vi "MAIN - TLB` Springboard Tool.vi"() -> ()   [LabVIEW 2015, in "TLB` Springboard.lvlib"]
doc: "TLB Prime - Application Template 1.3.0.24\nNorm Kirchner, NI Systems Engineering - NI\nCopyright (c) 2014, NI"
uses:
  TLB` Springboard.lvlib
  Components/State Declaration.ctl
  Components/System Triggers.ctl
  <vilib>/Utility/error.llb/DialogTypeEnum.ctl
  <vilib>/NI/AMC/Read Termination Message.vi
  <vilib>/NI/AMC/Create Single Message.vi
  <vilib>/NI/AMC/Update Message Routing Info.vi
  <vilib>/NI/AMC/Create Multiple Messages.vi
  Components/TypeDef - SHIFTER - TLB` Springboard.ctl
  <vilib>/NI/AMC/Globals.vi
  <vilib>/NI/AMC/Send Message.vi
  Components/Dependencies.llb/TLB`_Dependencies.lvlib
  <vilib>/NI/AMC/AMC.lvlib
panel:
  in  "Tab Control":T1(tab)
  out "Application:All Libraries in Application Instance":string[](array[string])
  out "Owned Items[]":refnum<vi>[](array[refnum])
  out "Array 1":string[](array[string])
  out "Array 2":string[](array[string])
  out "size(s) 1":i32
  out "size(s) 2":i32
  out "size(s) 4":i32
  out "Array 3":string[](array[string])
  out "Array 4":string[](array[string])
  out "Array 6":string[](array[string])
  out "Array 5":string[](array[string])
  out "size(s) 6":i32
  in  "Library Path":path=path "C:/Repositories/TLB-Prime/Source/TLB' Template 2/TLB` Template/TLB` Template.lvlib"
  in  "Add to Project":u16(ring) items=["< Create In New Project... >"]
  in  "Cancel":bool
  in  "Build":bool
  in  "New TLB Name":string="TEST"
  in  "Destination Folder":path=path "C:/Repositories/TLB-Prime/Stage"
  out "error out":errorcluster
  # "TLB` Springboard"
  # "Description"
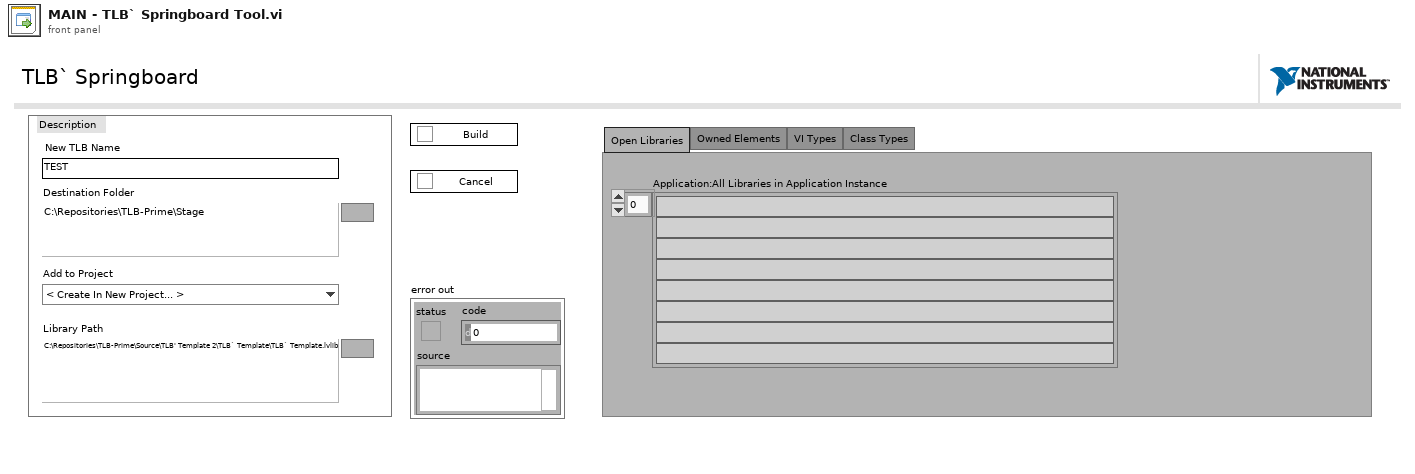
[diagram p1: front panel]
types:
  T1 = enum32{"Open Libraries", "Owned Elements", "VI Types", "Class Types"}
  T2 = typedef "TLB` Springboard.lvlib/System Triggers.ctl" = enum16{"<None>", "Create New", "Cache User Parameters", "Close Application"}
  T3 = typedef "TLB` Springboard.lvlib/State Declaration.ctl" = enum16{"<Startup>", "Idle", "Creating", "<Shutdown>"}
  T4 = enum16{"Clear SR", "Set Display", "Set Shifter", "Initialize Events", "Init Q"}
  T5 = typedef "TLB` Springboard.lvlib/TypeDef - SHIFTER - TLB` Springboard.ctl" = cluster{"State":T3, "User Data":cluster{"New TLB Name":string, "Destination Folder":path, "Project Selection":u16, "Library Path":path}, "Display Data":cluster{"Active Item Tag":string}, "User Parameter Controls":refnum<vi>[], "Framework Data":cluster{"Exit Event":T6, "Terminate Error":errorcluster}, "Private Data":cluster{"Projects In Memory":refnum<vi>[], "Build Complete":bool, "My Computer Ref":refnum<vi>, "Application Ref":refnum<vi>, "Library Ref":refnum<vi>, "Owned Items[]":refnum<vi>[]}}
  T6 = typedef "TLB` Springboard.lvlib/TLB`_Dependencies.lvlib/Exit Event Ref.ctl" = refnum<user-event>
  T7 = typedef "AMC.lvlib/Message Queue.ctl" = refnum<queue>
  T8 = typedef "DialogTypeEnum.ctl" = enum16{"no dialog", "OK message", "continue or stop message", "auto error handling dialog", "OK message + warnings", "continue/stop + warnings"}
  T9 = enum8{"Enabled", "Disabled", "Disabled and Grayed Out"}
  T10 = enum32{"Invalid", "Standard", "Closed", "Hidden", "Minimized", "Maximized"}
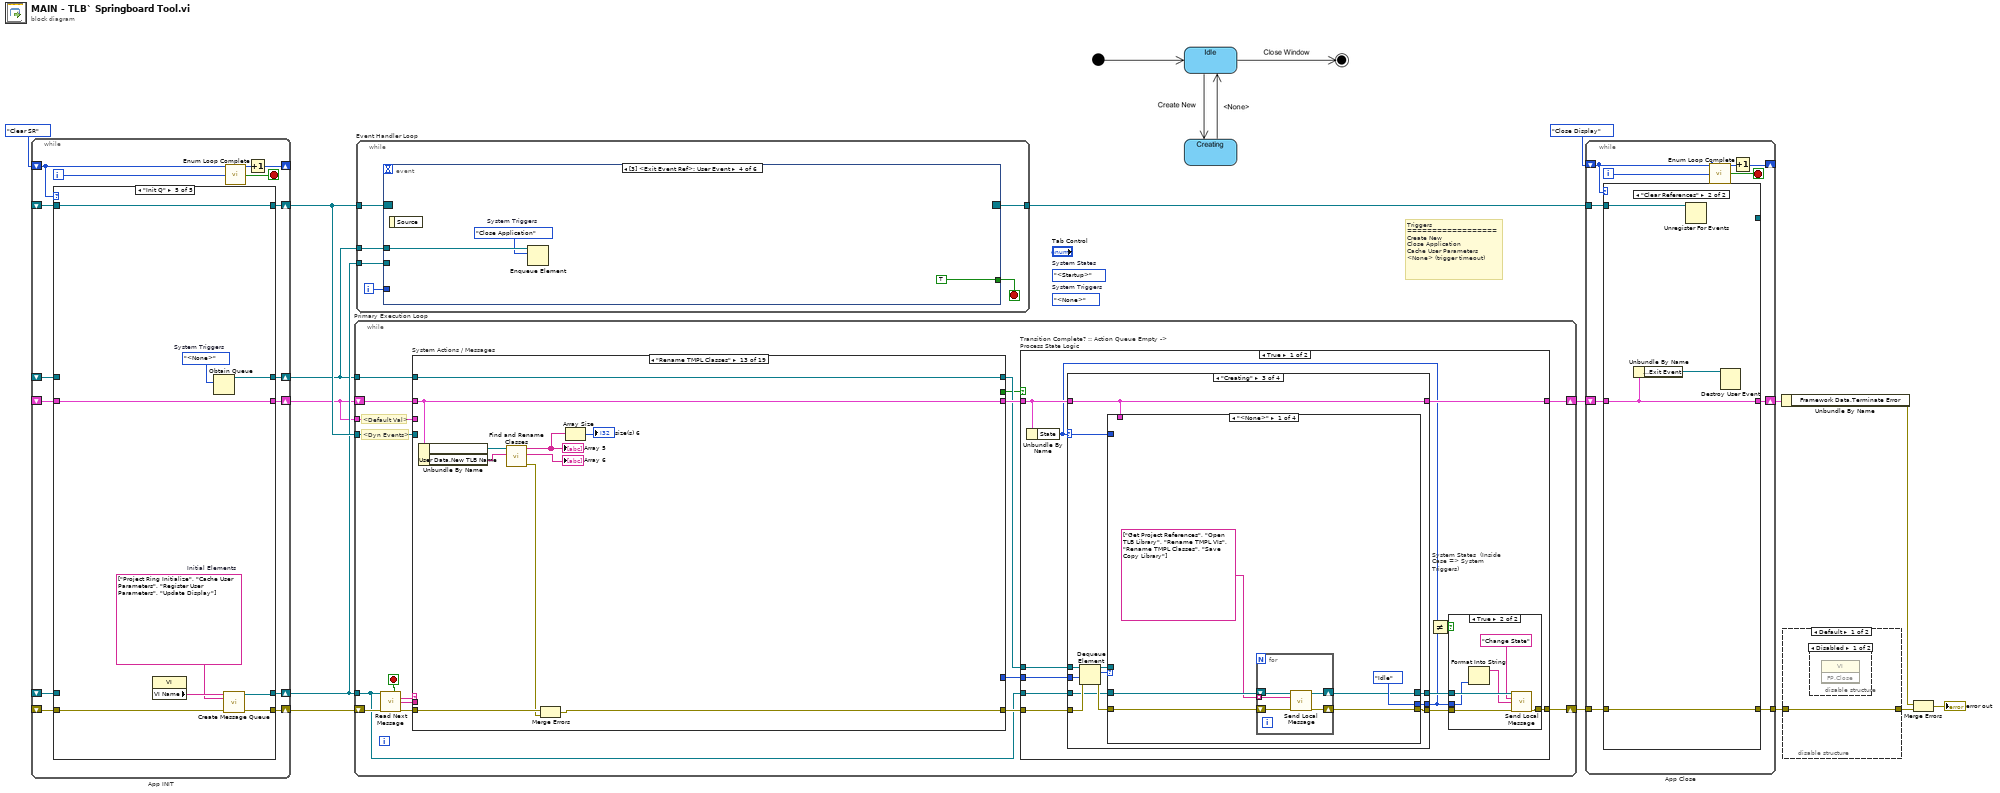
[diagram p0: block diagram]
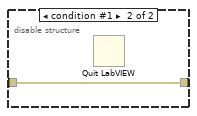
[diagram p3: hidden frame]
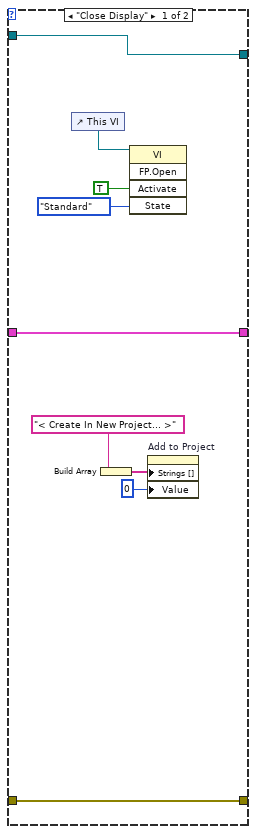
[diagram p4: hidden frame]
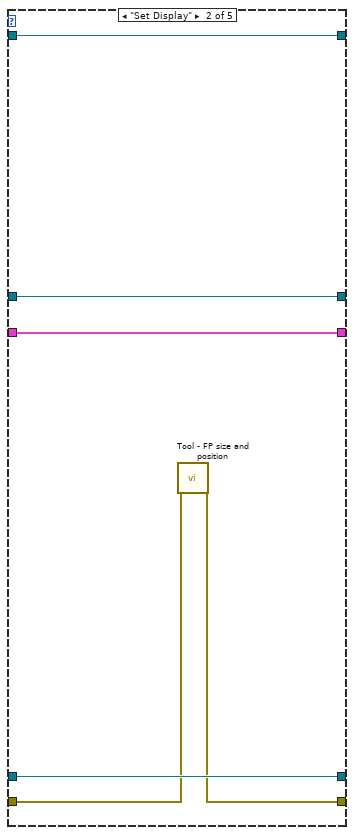
[diagram p6: hidden frame]
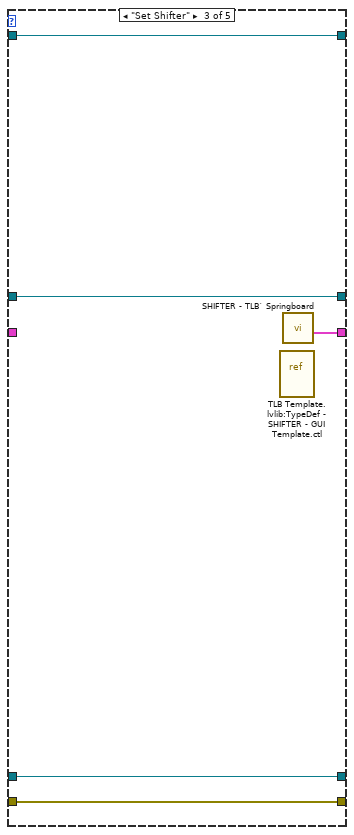
[diagram p7: hidden frame]
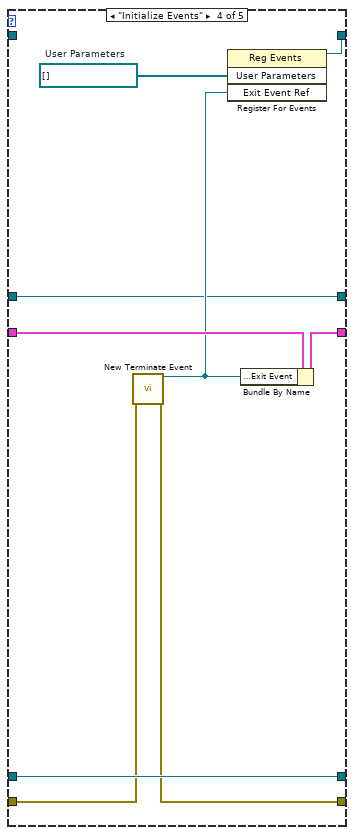
[diagram p8: hidden frame]
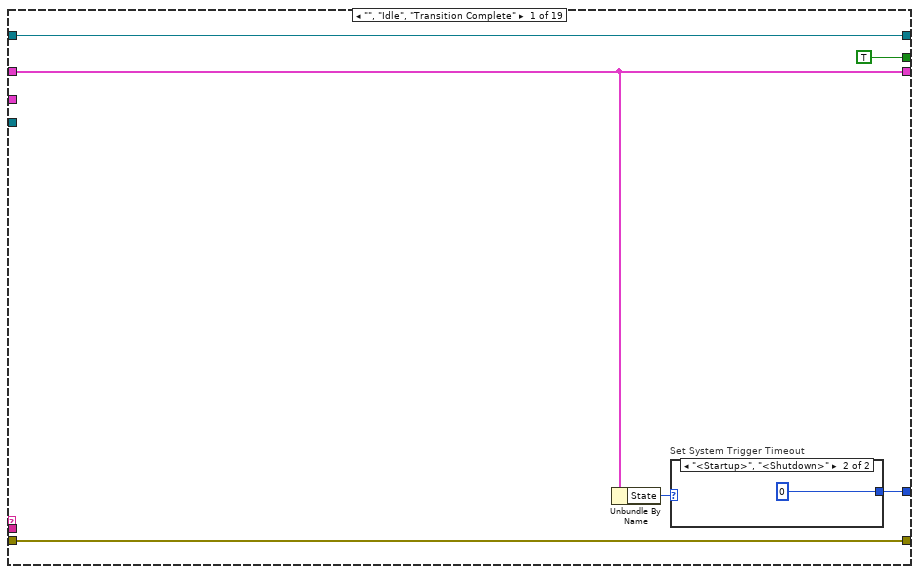
[diagram p9: hidden frame]
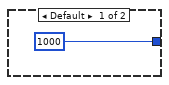
[diagram p10: hidden frame]
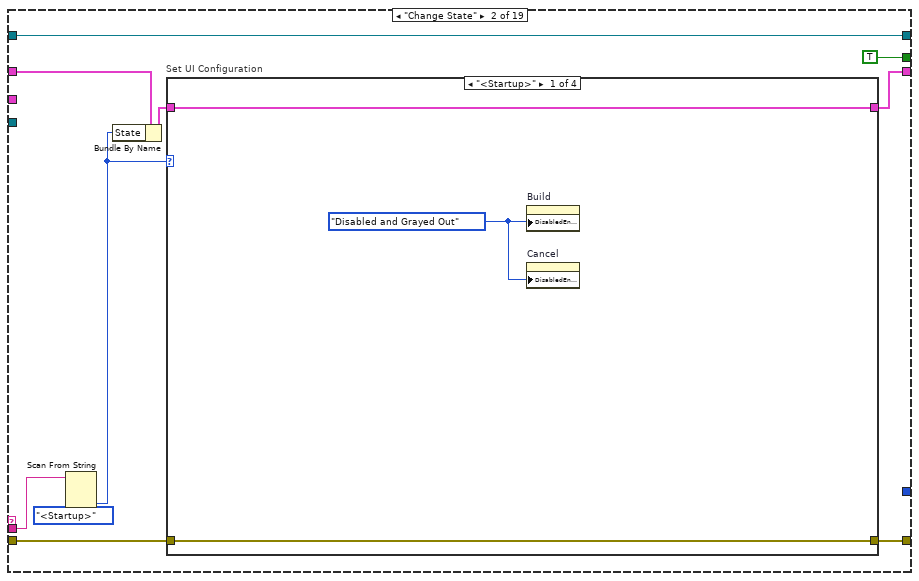
[diagram p11: hidden frame]
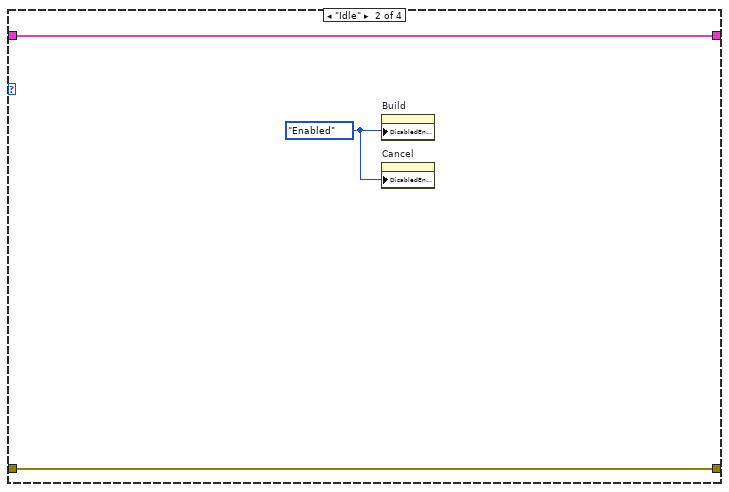
[diagram p12: hidden frame]
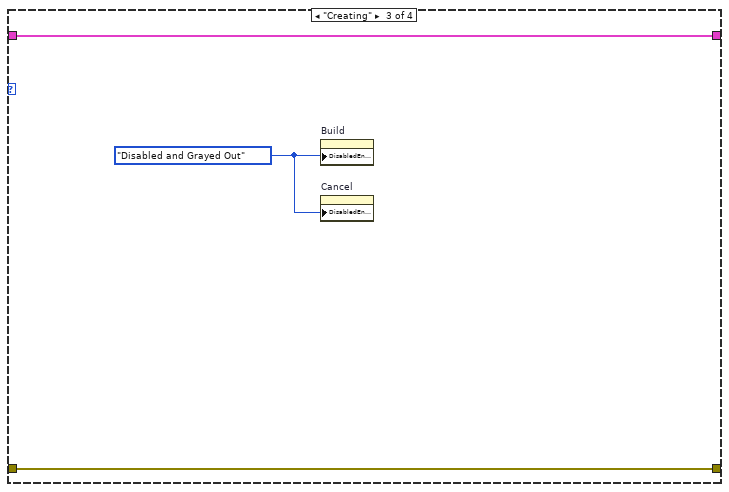
[diagram p13: hidden frame]
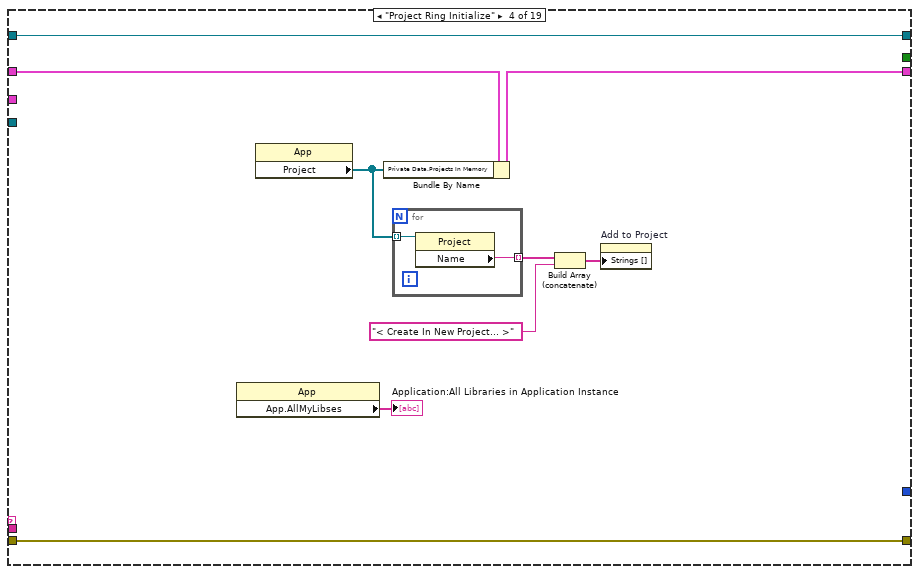
[diagram p16: hidden frame]
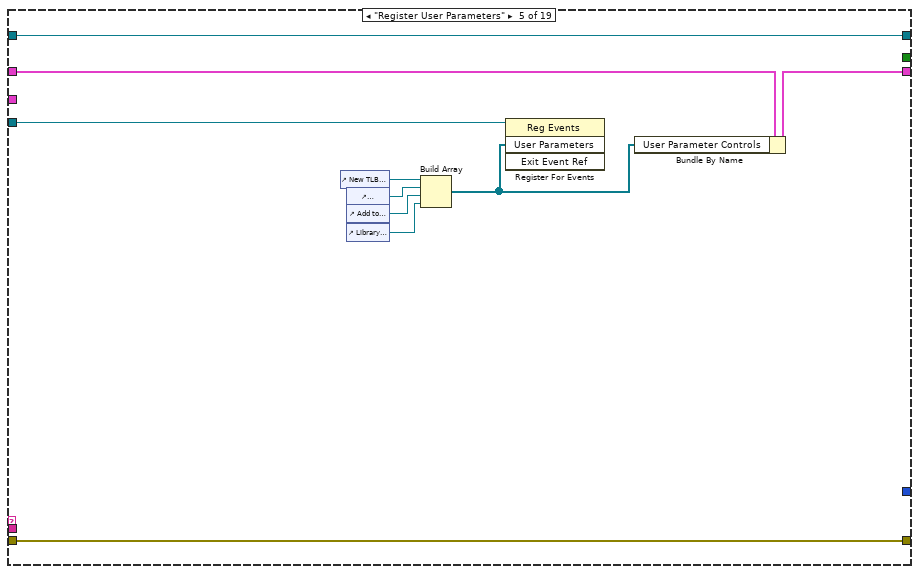
[diagram p17: hidden frame]
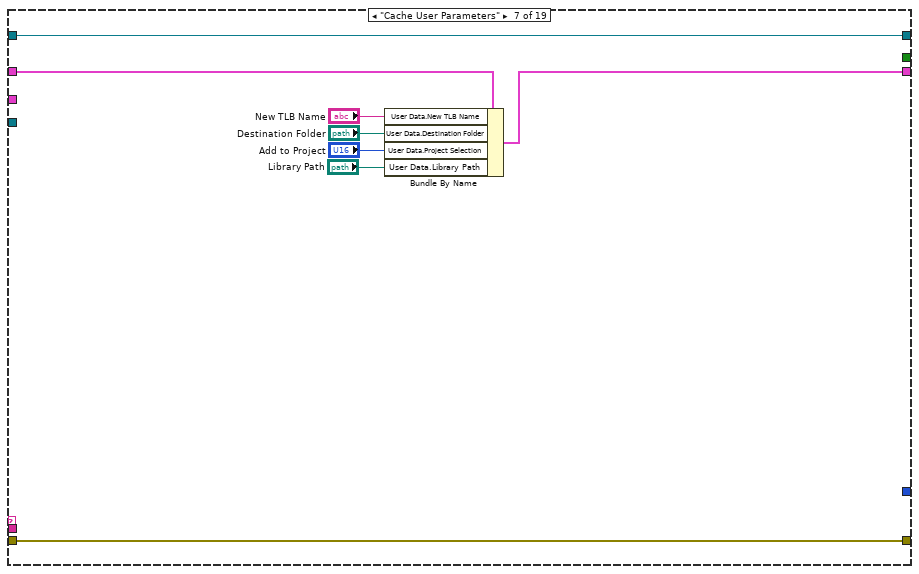
[diagram p19: hidden frame]
diagram:
  (unwired) System_Triggers."<None>"  # System Triggers
  (unwired) State_Declaration."<Startup>"  # System States
  # "Triggers\n==================\nCreate New\nClose Application\nCache User Parameters\n<None> (trigger timeout)"
  n1 = while "App INIT" {
    shift-right: [w23] -> _
    shift-left: T4."Clear SR" -> [w18]
    shift-right: [w29] -> w9
    shift-left: _ -> [w22]
    shift-right: [w26] -> w8
    shift-left: _ -> [w21]
    shift-right: [w28] -> w11
    shift-left: _ -> [w20]
    shift-right: [w27] -> w1
    shift-left: _ -> [w19]
    shift-right: [w17] -> w2
    shift-left: _ -> [w16]
    i -> [w24]
    stop <- w25 stop-if-true
    n2 = case shown="\"Init Q\"" w18 {
      tunnel: [_ w33 w40 w49 w55] -> w29
      tunnel: [_ w31 w39 w42 w53] -> w26
      tunnel: [_ w35 w36 w46 w57] -> w27
      tunnel: [_ w34 w38 w45 w58] -> w28
      tunnel: w22 -> [_ w33 w40 w49 _]
      tunnel: w21 -> [_ w32 w39 w43 w54]
      tunnel: w20 -> [_ w34 w38 _ w58]
      tunnel: w19 -> [_ w35 _ w47 w57]
      tunnel: [_ w30 w37 w41 w51] -> w17
      tunnel: w16 -> [_ w30 w37 w41 _]
      frame "Clear SR" {
      }
      frame "Set Display" {
        n3 = call "Tool - FP size and position.vi"("error in (no error)"=w32) -> ("error out"=w31:errorcluster)  [unwired: 7 in, 11 out]
      }
      frame "Set Shifter" {
        n4 = vi-ref "TLB Template.lvlib:TypeDef - SHIFTER - GUI Template.ctl"() -> ()  [unwired: 1 out]
        n5 = call "SHIFTER - TLB` Springboard.vi"() -> ("SHIFTER DATA"=w36:T5)  [unwired: 15 in]
      }
      frame "Initialize Events" {
        w48 = refnum<vi>[] []  # User Parameters
        n6 = call "New Terminate Event.vi"("error in (no error)"=w43) -> ("Exit Event Ref"=w44:T6, "error out"=w42:errorcluster)  [unwired: 13 in]
        n7 = register-events(w48, w44) -> (reference out=w45:refnum<event-registration>)  [unwired: 2 in, 1 out]
        n8 = Bundle By Name(cluster=w47, "Framework Data.Exit Event"=w44) -> (w46:T5)
      }
      frame "Init Q" {
        w50 = System_Triggers."<None>"  # System Triggers
        w52 = string[] ["Project Ring Initialize", "Cache User Parameters", "Register User Parameters", "Update Display"]  # Initial Elements
        n9 = property class="VI"() -> ("VI Name"=w56:string)  [unwired: 2 in, 2 out]
        n10 = Obtain Queue(element data type=w50) -> (queue out=w51:refnum<queue>)  [unwired: 4 in, 2 out]
        n11 = call <vilib>:"Create Message Queue.vi"("message queue name"=w56, "initial message names"=w52, "error in"=w54) -> ("message queue out"=w55:T7, "error out"=w53:errorcluster)  [unwired: 11 in]
      }
    }
    n12 = call "Enum Loop Complete.vi"("Current State Enum"=w18, "Itteration"=w24) -> ("Loop Complete?"=w25:bool)  [unwired: 13 out]
    n13 = Increment(x=w18) -> (x+1=w23:T4)
  }
  n14 = while "Primary Execution Loop" {
    shift-right: [w65] -> w15
    shift-left: w8 -> [w72]
    shift-right: [w68] -> w14
    shift-left: w1 -> [w75]
    tunnel: w1 -> [w74]
    tunnel: w9 -> [w63]
    tunnel: w11 -> [w73]
    tunnel: w2 -> [w64]
    stop <- w70 stop-if-true
    # "<Dyn Events>"
    # "<Default Val>"
    n15 = call <vilib>:"Read Next Message.vi"("message queue in"=w63, "error in"=w72) -> ("exit process?"=w70:bool, "message name"=w69:string, "message value"=w60:string, "error out"=w71:errorcluster)  [unwired: 6 in, 4 out]
    n16 = case "System Actions / Messages" shown="\"Rename TMPL Classes\"" w69 {
      selector: w69 -> [_ _ _ _ _ _ _ _ _ _ _ _ _ _ _ _ _ _ w282]
      tunnel: [w81 w88 w107 w114 w128 w131 w137 w142 w145 w157 w177 w184 w195 w220 w245 w250 w272 w276 w286] -> w66
      tunnel: w71 -> [w81 w87 w107 w114 w128 w131 w137 w142 w145 w157 w178 w192 w202 w224 w245 w251 w272 w275 w287]
      tunnel: w75 -> [w76 w84 w106 w116 w127 w130 w139 w141 w144 w150 w176 w187 w198 w219 w244 w248 w271 w279 w288]
      tunnel: w74 -> [_ _ _ _ _ _ _ _ _ _ _ _ _ _ _ _ _ _ _]
      tunnel: [w76 w86 w106 w111 w126 w130 w138 w141 w144 w148 w172 w187 w198 w218 w244 w249 w271 w279 w288] -> w67
      tunnel: [w77 _ _ _ _ _ _ _ _ _ _ _ _ _ _ _ _ _ _] -> w59
      tunnel: w73 -> [_ _ _ _ w125 _ _ _ _ _ _ _ _ _ _ _ _ _ _]
      tunnel: [w79 w92 w105 w115 w124 w129 w136 w140 w143 w156 w179 w191 w201 w225 w243 w246 w270 w273 w280] -> w62
      tunnel: w64 -> [w79 w92 w105 w115 w124 w129 w136 w140 w143 w156 w179 w191 w201 w225 w243 w246 w270 w273 w280]
      tunnel: [TRUE TRUE _ _ _ _ _ _ _ _ _ _ _ _ _ _ _ _ _] -> w61
      tunnel: w60 -> [_ w91 _ _ _ _ _ _ _ _ _ _ _ _ _ _ _ _ _]
      frame "", "Idle", "Transition Complete" {
        n17 = Unbundle By Name(w76) -> ("State"=w78:T3)
        n18 = case "Set System Trigger Timeout" shown="\"<Startup>\", \"<Shutdown>\"" w78 {
          tunnel: [1000 0] -> w77
          frame Default {
          }
          frame "<Startup>", "<Shutdown>" {
          }
        }
      }
      frame "Change State" {
        n19 = Scan From String(input string=w91, default 1=State_Declaration."<Startup>" ("State")) -> (output 1=w89:T3)  [unwired: 3 in, 3 out]
        n20 = Bundle By Name(cluster=w84, "State"=w89) -> (w85:T5)
        n21 = case "Set UI Configuration" shown="\"<Startup>\"" w89 {
          tunnel: [w95 w99 w102 w104] -> w88
          tunnel: w87 -> [w95 w99 w102 w104]
          tunnel: [w96 w98 w101 w103] -> w86
          tunnel: w85 -> [w96 w98 w101 w103]
          frame "<Startup>" {
            w94 = T9."Disabled and Grayed Out" ("Disabled")
            n22 = property on="Build" class="Bool"("DisabledEnum"=w94) -> ()  [unwired: 2 in, 2 out]
            n23 = property on="Cancel" class="Bool"("DisabledEnum"=w94) -> ()  [unwired: 2 in, 2 out]
          }
          frame "Idle" {
            w97 = T9."Enabled" ("Disabled")
            n24 = property on="Build" class="Bool"("DisabledEnum"=w97) -> ()  [unwired: 2 in, 2 out]
            n25 = property on="Cancel" class="Bool"("DisabledEnum"=w97) -> ()  [unwired: 2 in, 2 out]
          }
          frame "Creating" {
            w100 = T9."Disabled and Grayed Out" ("Disabled")
            n26 = property on="Build" class="Bool"("DisabledEnum"=w100) -> ()  [unwired: 2 in, 2 out]
            n27 = property on="Cancel" class="Bool"("DisabledEnum"=w100) -> ()  [unwired: 2 in, 2 out]
          }
          frame "<Shutdown>" {
          }
        }
      }
      frame "/***********Initialize***********/" {
      }
      frame "Project Ring Initialize" {
        n28 = property class="App"() -> ("App.AllMyLibses"=→"Application:All Libraries in Application Instance":string[])  [unwired: 2 in, 2 out]
        n29 = property class="App"() -> ("Project"=w110:refnum<vi>[])  [unwired: 2 in, 2 out]
        n30 = Bundle By Name(cluster=w116, "Private Data.Projects In Memory"=w110) -> (w111:T5)
        n31 = for {
          tunnel: w110 -> [w118] mode=indexing
          tunnel: [w117] -> w113 mode=indexing
          n32 = property class="Project"(reference=w118) -> ("Name"=w117:string)  [unwired: 1 in, 2 out]
        }
        n33 = Build Array (concatenate)(w113, "< Create In New Project... >") -> (w109:string[])
        n34 = property on="Add to Project" class="Ring (strict)"("Strings []"=w109) -> ()  [unwired: 2 in, 2 out]
      }
      frame "Register User Parameters" {
        n35 = control-ref of="New TLB Name"() -> (w122:refnum<vi>)
        n36 = control-ref of="Destination Folder"() -> (w120:refnum<vi>)
        n37 = control-ref of="Add to Project"() -> (w121:refnum<vi>)
        n38 = control-ref of="Library Path"() -> (w119:refnum<vi>)
        n39 = Build Array(w122, w120, w121, w119) -> (w123:refnum<vi>[])
        n40 = register-events(reference=w125, w123) -> ()  [unwired: 2 in, 2 out]
        n41 = Bundle By Name(cluster=w127, "User Parameter Controls"=w123) -> (w126:T5)
      }
      frame "/*******Display Updates******/" {
      }
      frame "Cache User Parameters" {
        n42 = Bundle By Name(cluster=w139, "User Data.New TLB Name"="New TLB Name", "User Data.Destination Folder"="Destination Folder", "User Data.Project Selection"="Add to Project", "User Data.Library Path"="Library Path") -> (w138:T5)
      }
      frame "Update Display" {
      }
      frame "/******Primary Execution*****/" {
      }
      frame "Get Project References" {
        n43 = Unbundle By Name(w150) -> ("Private Data.Projects In Memory"=w153:refnum<vi>[], "User Data.Project Selection"=w155:u16)
        n44 = To Long Integer(number=w155) -> (32bit integer=w151:i32)
        n45 = Array Size(array=w153) -> (size(s)=w154:i32)
        n46 = Less?(x=w151, y=w154) -> (x < y?=w152:bool)
        n47 = case shown="True" w152 {
          tunnel: w151 -> [_ w162]
          tunnel: w153 -> [_ w161]
          tunnel: [w158 w160] -> w149
          frame False {
            n48 = invoke class="App" method="Project.New"() -> ("Project:New"=w159:refnum<vi>)  [unwired: 3 in, 2 out]
            n49 = invoke class="Project" method="Open Window"(reference=w159) -> (reference out=w158:refnum<vi>)  [unwired: 2 in, 2 out]
          }
          frame True {
            n50 = Index Array(array=w161, index=w162) -> (element=w160:refnum<vi>)
          }
        }
        n51 = property class="Project"(reference=w149) -> ("My Computer"=w147:refnum<vi>, "App Ref"=w146:refnum<vi>)  [unwired: 1 in, 2 out]
        n52 = Bundle By Name(cluster=w150, "Private Data.My Computer Ref"=w147, "Private Data.Application Ref"=w146) -> (w148:T5)
      }
      frame "Open TLB Library" {
        n53 = Unbundle By Name(w176) -> ("User Data.Library Path"=w174:path, "Private Data.Application Ref"=w173:refnum<vi>)
        n54 = call <vilib>:"Set Busy.vi"("error in (no error)"=w178) -> ("error out"=w175:errorcluster)  [unwired: 9 in, 1 out]
        n55 = invoke class="App" method="Library.Open"(reference=w173, error in=w175, "path"=w174) -> (error out=w171:errorcluster, "Open Library"=w170:refnum<vi>)  [unwired: 1 in, 2 out]
        n56 = property class="Library"(reference=w170) -> ("Children[]"=w163:refnum<vi>[])  [unwired: 1 in, 2 out]
        n57 = call "Recursive Owned VIs List.vi"("Parent[]"=w163) -> ("Children[]"=w165:refnum<vi>[])  [unwired: 10 in]
        n58 = Build Array (concatenate)(w163, w165) -> (w164:refnum<vi>[])
        "Owned Items[]" <- w164
        n59 = Bundle By Name(cluster=w176, "Private Data.Library Ref"=w170, "Private Data.Owned Items[]"=w164) -> (w172:T5)
        n60 = Array Size(array=w164) -> (size(s)=→"size(s) 1":i32)
        n61 = for {
          tunnel: w164 -> [w182] mode=indexing
          tunnel: [w181] -> w169 mode=indexing
          tunnel: [w180] -> w166 mode=indexing
          n62 = property class="ProjectItem"(reference=w182) -> ("Type String"=w181:string, "Display Name"=w180:string)  [unwired: 1 in, 2 out]
        }
        "Array 1" <- w169
        "Array 2" <- w166
        n63 = call <vilib>:"Unset Busy.vi"("error in (no error)"=w171) -> ("error out"=w177:errorcluster)  [unwired: 10 in]
        n64 = Array Size(array=w166) -> (size(s)=→"size(s) 2":i32)
      }
      frame "Rename TMPL VIs" {
        n65 = Unbundle By Name(w187) -> ("Private Data.Owned Items[]"=w186:refnum<vi>[], "User Data.New TLB Name"=w185:string)
        n66 = call "Find and Rename VIs.vi"("New TLB Name"=w185, "Owned Items[]"=w186) -> ("error out"=w183:errorcluster, "Array 2"=→"Array 4":string[], "Array"=w188:string[])  [unwired: 7 in]
        "Array 3" <- w188
        n67 = Merge Errors(w192, w183) -> (w184:errorcluster)
        n68 = Array Size(array=w188) -> (size(s)=→"size(s) 4":i32)
      }
      frame "Rename TMPL Classes" {
        n69 = Unbundle By Name(w198) -> ("Private Data.Owned Items[]"=w197:refnum<vi>[], "User Data.New TLB Name"=w196:string)
        n70 = call "Find and Rename Classes.vi"("New TLB Name"=w196, "Owned Items[]"=w197) -> ("error out"=w194:errorcluster, "Array 2"=→"Array 6":string[], "Array"=w199:string[])  [unwired: 7 in]
        "Array 5" <- w199
        n71 = Merge Errors(w202, w194) -> (w195:errorcluster)
        n72 = Array Size(array=w199) -> (size(s)=→"size(s) 6":i32)
      }
      frame "Save Copy Library" {
        n73 = call <vilib>:"Set Busy.vi"("error in (no error)"=w224) -> ("error out"=w204:errorcluster)  [unwired: 9 in, 1 out]
        n74 = Unbundle By Name(w219) -> ("Private Data.Library Ref"=w203:refnum<vi>, "Private Data.My Computer Ref"=w206:refnum<vi>, "Private Data.Application Ref"=w205:refnum<vi>)
        n75 = Unbundle By Name(w219) -> ("User Data.Destination Folder"=w208:path, "User Data.New TLB Name"=w207:string)
        n76 = disable-structure shown="Disabled" {
          disable-tunnel: [w238 w241] -> w216
          disable-tunnel: [w237 _] -> w214
          disable-tunnel: [w236 w242] -> w213
          disable-tunnel: [w235 w240] -> w212
          disable-tunnel: w208 -> [w233 _]
          disable-tunnel: w207 -> [w232 _]
          disable-tunnel: w206 -> [w231 w242]
          disable-tunnel: w204 -> [w230 w241]
          disable-tunnel: w203 -> [w229 w240]
          frame Disabled {
            n77 = invoke class="Library" method="Save a Copy"(reference=w229, error in=w230, "Path"=w233, "New Name"=w232) -> (reference out=w235:refnum<vi>, error out=w239:errorcluster, "New Lib Path"=w234:path)  [unwired: 2 in, 3 out]
            n78 = invoke class="TargetItem" method="AddFile"(reference=w231, error in=w239, "Path"=w234) -> (reference out=w236:refnum<vi>, error out=w238:errorcluster, "AddFile"=w237:refnum<vi>)  [unwired: 1 in, 1 out]
          }
          frame Enabled {
          }
        }
        n79 = Close Reference(reference=w212, error in (no error)=w216) -> (error out=w211:errorcluster)
        n80 = Close Reference(reference=w205, error in (no error)=w211) -> (error out=w210:errorcluster)
        n81 = disable-structure shown="Disabled" {
          disable-tunnel: [w228 _] -> w215
          disable-tunnel: w214 -> [w227 _]
          disable-tunnel: w210 -> [w226 _]
          frame Disabled {
            n82 = Close Reference(reference=w227, error in (no error)=w226) -> (error out=w228:errorcluster)
          }
          frame Enabled {
          }
        }
        n83 = VI Library() -> (path=w223:path)
        n84 = Close Reference(reference=w213, error in (no error)=w215) -> (error out=w209:errorcluster)
        n85 = Unbundle By Name(w209) -> ("status"=w221:bool)
        n86 = call <vilib>:"Unset Busy.vi"("error in (no error)"=w209) -> ("error out"=w220:errorcluster)  [unwired: 10 in]
        n87 = Not(x=w221) -> (.not. x?=w217:bool)
        n88 = Bundle By Name(cluster=w219, "Private Data.Build Complete"=w217) -> (w218:T5)
        n89 = Build Path(base path=w223, name or relative path="..\\project\\_TLB`\\TLB` Template\\TLB` Template.lvlib") -> ()  [unwired: 1 out]
      }
      frame "/**********Shutdown*********/" {
      }
      frame "Error" {
        n90 = Unbundle By Name(w248) -> ("State"=w247:T3)
        n91 = case shown="Default" w247 {
          tunnel: w251 -> [w259]
          tunnel: [w258] -> w250
          tunnel: w248 -> [w255]
          tunnel: [w254] -> w249
          tunnel: w246 -> [w252]
          frame Default {
            n92 = call <vilib>:"General Error Handler CORE.vi"("type of dialog (OK msg:1)"=DialogTypeEnum."auto error handling dialog", "error in (no error)"=w259) -> ("stop event propagated"=w257:bool, "error out"=w253:errorcluster)  [unwired: 12 out]
            n93 = case "User Chose to Stop and Not Continue\nFALSE = Continue: CLEAR ERRORS" shown="True" w257 {
              tunnel: [w260 w264] -> w258
              tunnel: w253 -> [w261 w267]
              tunnel: w255 -> [w262 w269]
              tunnel: [w262 w268] -> w254
              tunnel: w252 -> [_ w265]
              frame False {
                n94 = call <vilib>:"Clear Errors.vi"("error in (no error)"=w261) -> ("error out"=w260:errorcluster)  [unwired: 1 in, 5 out]
              }
              frame True {
                n95 = call <vilib>:"Clear Errors.vi"("error in (no error)"=w267) -> ("error out"=w263:errorcluster)  [unwired: 1 in, 5 out]
                n96 = Bundle By Name(cluster=w269, "Framework Data.Terminate Error"=w267) -> (w268:T5)
                n97 = Enqueue Element(queue=w265, element=System_Triggers."Close Application", error in (no error)=w263) -> (error out=w264:errorcluster)  [unwired: 1 in, 2 out]
              }
            }
          }
        }
      }
      frame "Close Window" {
      }
      frame "Exit" {
        w274 = refnum<class> refnum  # event data
        # "Don't wire 'Error In'\nMust Execute Regardless"
        n98 = Unbundle By Name(w279) -> ("Framework Data.Exit Event"=w278:T6)
        n99 = Generate User Event(user event=w278, event data cluster=w274) -> (error out=w277:errorcluster)  [unwired: 2 in, 1 out]
        n100 = Merge Errors(w277, w275) -> (w276:errorcluster)
      }
      frame Default {
        w284 = 1 items=["No error", "Argument error", "Memory is full", "Out of zone", "End of file", "File already open", "Generic file I/O error", "File not found", "File permission error", "Disk is full", "Duplicate path", "Too many files open", "System feature not enabled", "Resource file not found", "Cannot add resource", "Resource not found", "Image not found", "Image memory error", "Pen does not exist", "Config type invalid", "Config token not found", "Config parse error", "Config memory error", "Bad external code format", "Bad external code offset", "External code not present", "Null window", "Destroy window error", "Null menu", "Print aborted", "Bad print record", "Print driver error", "Windows error during printing", "Memory error during printing", "Print dialog error", "Generic print error", "Invalid device refnum", "Device not found", "Device parameter error", "Device unit error", "Cannot open device", "Device call aborted", "Generic error", "Cancelled by user", "Object ID too low", "Object ID too high", "Object not in heap", "Unknown heap", "Unknown object (invalid DefProc)", "Unknown object (DefProc not in table)", "Message out of range", "Invalid (null) method", "Unknown message", "Manager call not supported", "Bad address", "Network operation in progress", "Network operation timed out", "Connection is busy", "Network attribute not supported", "Network error", "Address in use", "System out of memory", "Connection aborted", "Connection refused", "Not connected", "Already connected", "Connection closed", "Initialization error (interapplication manager)", "Bad occurrence", "Wait on unbound occurrence handler", "Occurrence queue overflow", "Datalog type conflict", "Unused", "Unrecognized type (interapplication manager)", "Memory corrupt", "Failed to make temporary DLL", "Old CIN version", "Drag socket not found", "Failed to load drop-object", "Failed to register OLE object", "Failed to release OLE object", "Format specifier type mismatch", "Unknown format specifier", "Too few format specifiers", "Too many format specifiers", "Scan failed", "Newer CIN version", "Error converting to variant", "Runtime menu error", "Password tampered", "Variant attribute not found", "Incompatible variant data type", "Event data is not available", "Event Store is not present", "Occurrence is not found", "Event Queue is not created", "Event info is not available", "Refnum passed is NULL", "Error retrieving Class GUID", "Error retrieving CoClass GUID", "Error retrieving TypeLib GUID.", "Bad built application magic bytes.", "Specific driver is different from the specific driver associated with the Logical Name.", "There is no session opened to the class driver.", "Max Error", "MAX - Error with config objects", "MAX - Error loading configuration", "MAX - Group not supported"]
        w285 = TRUE  # status
        n101 = Format Into String(format string="DEVELOPER ERROR:\nImproper State Requested\n================\nState {%s} does not exist within this architecture\n\nCheck for spelling and case errors" ("source"), w282) -> (resulting string=w283:string)  [unwired: 2 in, 1 out]
        n102 = Bundle By Name(cluster=w287, "status"=w285, "code"=w284, "source"=w283) -> (w286:errorcluster)
      }
    }
    n103 = case "Transition Complete? :: Action Queue Empty -> Process State Logic" shown="True" w61 {
      tunnel: [w300 w419] -> w68
      tunnel: w67 -> [w290 w419]
      tunnel: w66 -> [w299 w418]
      tunnel: w63 -> [w298 _]
      tunnel: [w294 w418] -> w65
      tunnel: w62 -> [w297 _]
      tunnel: w59 -> [w291 _]
      frame True {
        n104 = Unbundle By Name(w290) -> ("State"=w289:T3)
        n105 = case "System States  (Inside Case => System Triggers)" shown="\"Creating\"" w289 {
          selector: w289 -> [_ w333 w363 _]
          tunnel: [w316 w332 w373 w409] -> w300
          tunnel: w290 -> [w316 w332 w373 w409]
          tunnel: w299 -> [w310 w337 w367 w403]
          tunnel: w298 -> [w308 w335 w365 w401]
          tunnel: [w315 w342 w372 w408] -> w295
          tunnel: w297 -> [w318 w331 w374 w411]
          tunnel: [w314 w341 w371 w407] -> w296
          tunnel: [w313 w340 w370 w406] -> w293
          tunnel: w291 -> [w312 w338 w368 w405]
          frame "<Startup>" {
            n106 = Dequeue Element(queue=w318, timeout in ms (-1)=w312, error in (no error)=w310) -> (queue out=w311:refnum<queue>, element=w317:T2, error out=w309:errorcluster)  [unwired: 1 out]
            n107 = case shown="\"<None>\", Default" w317 {
              tunnel: w316 -> [_]
              tunnel: [w319] -> w315
              tunnel: w309 -> [w322]
              tunnel: w308 -> [w323]
              tunnel: [w320] -> w314
              tunnel: [State_Declaration."Idle" ("State")] -> w313
              tunnel: w311 -> [_]
              frame "<None>", Default {
                n108 = for {
                  shift-right: [w328] -> w319
                  shift-left: w322 -> [w329]
                  shift-right: [w326] -> w320
                  shift-left: w323 -> [w327]
                  tunnel: string[] [] -> [w325] mode=indexing
                  n109 = call <vilib>:"Send Local Message.vi"("message queue in"=w327, "message name"=w325, "error in"=w329) -> ("message queue out"=w326:T7, "error out"=w328:errorcluster)  [unwired: 10 in, 1 out]
                }
              }
            }
          }
          frame "Idle" {
            n110 = Dequeue Element(queue=w331, timeout in ms (-1)=w338, error in (no error)=w337) -> (queue out=w334:refnum<queue>, element=w339:T2, error out=w336:errorcluster)  [unwired: 1 out]
            n111 = Unbundle By Name(w332) -> ()  [unwired: 1 out]
            n112 = case shown="\"Cache User Parameters\"" w339 {
              tunnel: w332 -> [_ _ _ _ _]
              tunnel: [w345 w349 w352 w355 w359] -> w342
              tunnel: w336 -> [w345 w349 w352 w355 w362]
              tunnel: w335 -> [w346 w348 w353 w356 w361]
              tunnel: [w346 w348 w353 w356 w360] -> w341
              tunnel: [State_Declaration."Idle" ("State") State_Declaration."Creating" ("State") State_Declaration."<Shutdown>" ("State") State_Declaration."Idle" ("State") w357] -> w340
              tunnel: w334 -> [_ _ _ _ _]
              tunnel: w333 -> [_ _ _ _ w357]
              frame "<None>" {
              }
              frame "Create New" {
              }
              frame "Close Application" {
              }
              frame Default {
              }
              frame "Cache User Parameters" {
                n113 = call <vilib>:"Send Local Message.vi"("message queue in"=w361, "message name"="Cache User Parameters" ("Message Name"), "error in"=w362) -> ("message queue out"=w360:T7, "error out"=w359:errorcluster)  [unwired: 10 in, 1 out]
              }
            }
            n114 = case shown="True" FALSE {
              tunnel: w331 -> [_ w343]
              frame False {
              }
              frame True {
                n115 = Enqueue Element(queue=w343, element=System_Triggers."Close Application" ("System Triggers")) -> ()  [unwired: 2 in, 3 out]
              }
            }
          }
          frame "Creating" {
            n116 = Dequeue Element(queue=w374, timeout in ms (-1)=w368, error in (no error)=w367) -> (queue out=w364:refnum<queue>, element=w369:T2, error out=w366:errorcluster)  [unwired: 1 out]
            n117 = case shown="\"<None>\"" w369 {
              tunnel: w373 -> [_ _ _ _]
              tunnel: [w378 w388 w392 w396] -> w372
              tunnel: w366 -> [w379 w391 w392 w397]
              tunnel: w365 -> [w377 w390 w393 w395]
              tunnel: [w376 w389 w393 w395] -> w371
              tunnel: [State_Declaration."Idle" ("State") w386 State_Declaration."Creating" ("State") State_Declaration."Idle" ("State")] -> w370
              tunnel: w364 -> [_ _ _ w399]
              tunnel: w363 -> [_ w386 _ _]
              frame "<None>" {
                n118 = for {
                  shift-right: [w384] -> w378
                  shift-left: w379 -> [w385]
                  shift-right: [w382] -> w376
                  shift-left: w377 -> [w383]
                  tunnel: string[] ["Get Project References", "Open TLB Library", "Rename TMPL VIs", "Rename TMPL Classes", "Save Copy Library"] -> [w381] mode=indexing
                  n119 = call <vilib>:"Send Local Message.vi"("message queue in"=w383, "message name"=w381, "error in"=w385) -> ("message queue out"=w382:T7, "error out"=w384:errorcluster)  [unwired: 10 in, 1 out]
                }
              }
              frame "Cache User Parameters" {
                n120 = call <vilib>:"Send Local Message.vi"("message queue in"=w390, "message name"="Cache User Parameters" ("Message Name"), "error in"=w391) -> ("message queue out"=w389:T7, "error out"=w388:errorcluster)  [unwired: 10 in, 1 out]
              }
              frame Default {
              }
              frame "Close Application" {
                n121 = Enqueue Element(queue=w399, element=System_Triggers."Close Application" ("System Triggers"), error in (no error)=w397) -> (error out=w396:errorcluster)  [unwired: 1 in, 2 out]
              }
            }
          }
          frame "<Shutdown>" {
            n122 = Dequeue Element(queue=w411, timeout in ms (-1)=w405, error in (no error)=w403) -> (queue out=w404:refnum<queue>, element=w410:T2, error out=w402:errorcluster)  [unwired: 1 out]
            n123 = case shown="\"<None>\", Default" w410 {
              tunnel: w409 -> [_]
              tunnel: [w412] -> w408
              tunnel: w402 -> [w414]
              tunnel: w401 -> [w415]
              tunnel: [w413] -> w407
              tunnel: [State_Declaration."<Shutdown>" ("State")] -> w406
              tunnel: w404 -> [_]
              frame "<None>", Default {
                n124 = call <vilib>:"Send Local Messages.vi"("message queue in"=w415, "message names"=string[] ["Exit"], "error in"=w414) -> ("message queue out"=w413:T7, "error out"=w412:errorcluster)  [unwired: 10 in, 1 out]
              }
            }
          }
        }
        n125 = Not Equal?(x=w289, y=w293) -> (x != y?=w292:bool)
        n126 = case shown="True" w292 {
          tunnel: w296 -> [_ w307]
          tunnel: w295 -> [w301 w306]
          tunnel: [w301 w305] -> w294
          tunnel: w293 -> [_ w303]
          frame False {
          }
          frame True {
            n127 = Format Into String(w303) -> (resulting string=w302:string)  [unwired: 3 in, 1 out]
            n128 = call <vilib>:"Send Local Message.vi"("message queue in"=w307, "message name"="Change State" ("Message Name"), "message value"=w302, "error in"=w306) -> ("error out"=w305:errorcluster)  [unwired: 9 in, 2 out]
          }
        }
      }
      frame False {
      }
    }
  }
  n129 = while "Event Handler Loop" {
    tunnel: w11 -> [w424]
    tunnel: w9 -> [w423]
    tunnel: [w422] -> w13
    tunnel: w2 -> [w420]
    i -> [w421]
    stop <- w425 stop-if-true
    n130 = event shown="[3] <Exit Event Ref>: User Event" {
      selector: w424 -> [_ _ _ _ _ _]
      dyn-events: [_ _ _ _ _ _] -> w422
      timeout: _ -> [_ _ _ _ _ _]
      tunnel: [_ _ _ TRUE ("NewVal") _ _] -> w425
      tunnel: w423 -> [_ _ _ _ _ _]
      tunnel: w421 -> [_ _ _ _ _ _]
      tunnel: w420 -> [w427 w430 _ w443 w447 w449]
      event Panel Close? {
        w428 = TRUE  # Discard?
        n131 = event-data() -> ()  [unwired: 2 out]
        n132 = Enqueue Element(queue=w427, element=System_Triggers."Close Application") -> ()  [unwired: 2 in, 3 out]
        n133 = event-data("Discard?"=w428) -> ()  [unwired: 1 in, 1 out]
      }
      event "Cancel": Value Change {
        n134 = event-data() -> ()  [unwired: 4 out]
        n135 = Enqueue Element(queue=w430, element=System_Triggers."Close Application") -> ()  [unwired: 2 in, 3 out]
      }
      event Mouse Down {
        n136 = event-data() -> ("Button"=w435:u16, "Mods"=w436:cluster{"Double Click":bool, "Menu Key":bool})  [unwired: 1 out]
        n137 = Unbundle By Name(w436) -> ("Double Click"=w432:bool)
        n138 = Equal?(x=u16 2, y=w435) -> (x = y?=w433:bool)
        n139 = And(x=w433, y=w432) -> (x .and. y?=w431:bool)
        n140 = case "Toggle Menu Visibility :: double RIGHT click on logo" shown="True" w431 {
          frame False {
          }
          frame True {
            n141 = property class="VI"() -> (reference out=w441:refnum<vi>, "TB.Visible"=w439:bool, "Front Panel.ShowMenuBar"=w438:bool)  [unwired: 2 in, 1 out]
            n142 = Not(x=w439) -> (.not. x?=w440:bool)
            n143 = Not(x=w438) -> (.not. x?=w437:bool)
            n144 = property class="VI"(reference=w441, "TB.Visible"=w440, "Front Panel.ShowMenuBar"=w437) -> ()  [unwired: 1 in, 2 out]
          }
        }
      }
      event User Event {
        w442 = System_Triggers."Close Application"  # System Triggers
        n145 = event-data() -> ()  [unwired: 2 out]
        n146 = Enqueue Element(queue=w443, element=w442) -> ()  [unwired: 2 in, 3 out]
      }
      event Value Change {
        n147 = event-data() -> ()  [unwired: 2 out]
        n148 = Enqueue Element(queue=w447, element=System_Triggers."Cache User Parameters") -> (queue out=w446:refnum<queue>)  [unwired: 2 in, 2 out]
        n149 = event "use this event case to register a SPEICIFIC 'User Parameter' for a SPECIFIC action" shown="[0] Timeout" {
          selector: _ -> [_]
          dyn-events: _ -> [_]
          timeout: 0 -> [_]
          tunnel: w446 -> [_]
          event Timeout {
            n150 = event-data() -> ()  [unwired: 1 in, 1 out]
          }
        }
      }
      event "Build": Value Change {
        n151 = event-data() -> ()  [unwired: 4 out]
        n152 = Enqueue Element(queue=w449, element=System_Triggers."Create New") -> ()  [unwired: 2 in, 3 out]
      }
    }
  }
  n153 = while "App Close" {
    shift-right: [w457] -> _
    shift-left: enum16{"Close Display", "Clear References"}."Close Display" -> [w456]
    tunnel: w13 -> [w454]
    tunnel: w15 -> [w455]
    tunnel: [w452] -> w7
    shift-right: [w451] -> w5
    shift-left: w14 -> [w453]
    i -> [w458]
    stop <- w459 stop-if-true
    n154 = case shown="\"Clear References\"" w456 {
      tunnel: [w467 w472] -> w452
      tunnel: [w466 w471] -> w451
      tunnel: [w468 _] -> _
      tunnel: w455 -> [w467 w472]
      tunnel: w454 -> [w468 w469]
      tunnel: w453 -> [w466 w471]
      frame "Close Display" {
        n155 = control-ref of="This VI"() -> (w460:refnum<vi>)
        n156 = Build Array("< Create In New Project... >") -> (w465:string[])
        n157 = invoke class="VI" method="FP.Open"(reference=w460, "Activate"=TRUE ("Activate?"), "State"=T10."Standard") -> ()  [unwired: 2 in, 5 out]
        n158 = property on="Add to Project" class="Ring (strict)"("Strings []"=w465, "Value"=u16 0) -> ()  [unwired: 2 in, 2 out]
      }
      frame "Clear References" {
        n159 = Unbundle By Name(w471) -> ("Framework Data.Exit Event"=w470:T6)
        n160 = Unregister For Events(event registration refnum=w469) -> ()  [unwired: 1 in, 1 out]
        n161 = Destroy User Event(user event=w470) -> ()  [unwired: 1 in, 1 out]
      }
    }
    n162 = call "Enum Loop Complete.vi"("Current State Enum"=w456, "Itteration"=w458) -> ("Loop Complete?"=w459:bool)  [unwired: 13 out]
    n163 = Increment(x=w456) -> (x+1=w457:enum16{"Close Display", "Clear References"})
  }
  n164 = Unbundle By Name(w5) -> ("Framework Data.Terminate Error"=w3:errorcluster)
  n165 = disable-structure shown="Default" {
    disable-tunnel: [w473 w474] -> w4
    disable-tunnel: w7 -> [w473 w474]
    frame condition #0 (active) {
      n166 = disable-structure shown="Disabled" {
        frame Disabled {
          n167 = invoke class="VI" method="FP.Close"() -> ()  [unwired: 3 in, 3 out]
        }
        frame Enabled {
        }
      }
    }
    frame condition #1 {
      n168 = Quit LabVIEW() -> ()  [unwired: 1 in]
    }
  }
  n169 = Merge Errors(w3, w4) -> (→"error out":errorcluster)
